vi "APPLICATION_Template.vi"(8 "error in":errorcluster) -> (0 "error out":errorcluster, 3 "Cancelled":bool)   [LabVIEW 2016]
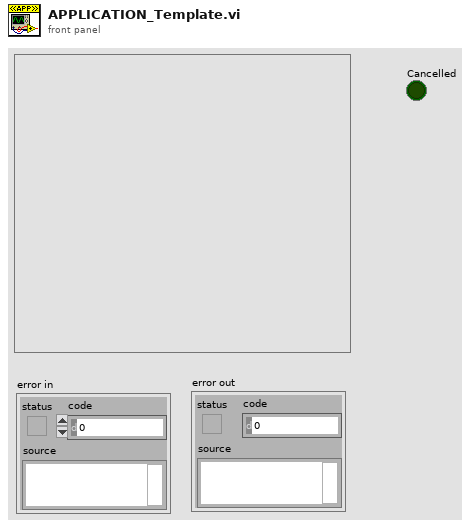
[diagram p1: front panel]
types:
  T1 = cluster{"Counter":i32, "Text":string, "Cancelled":bool}
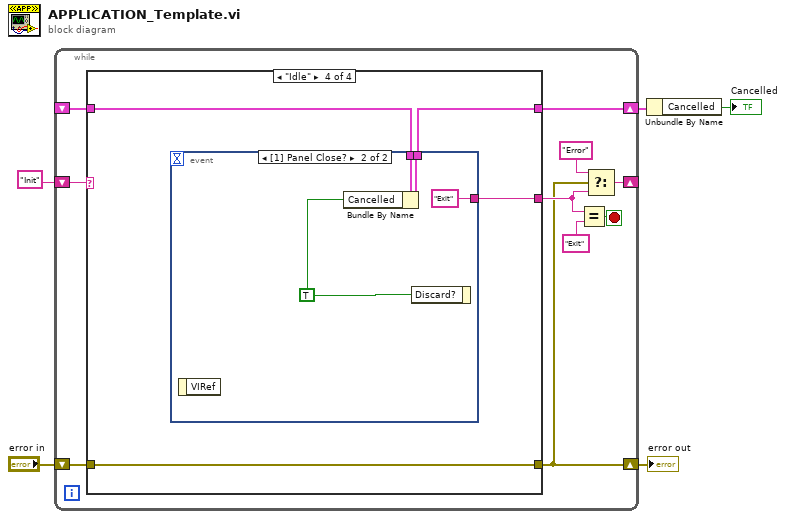
[diagram p0: block diagram]
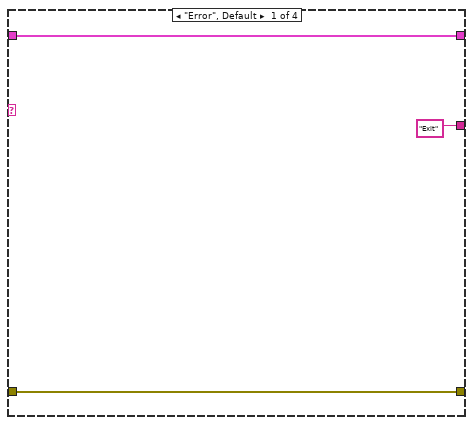
[diagram p2: hidden frame]
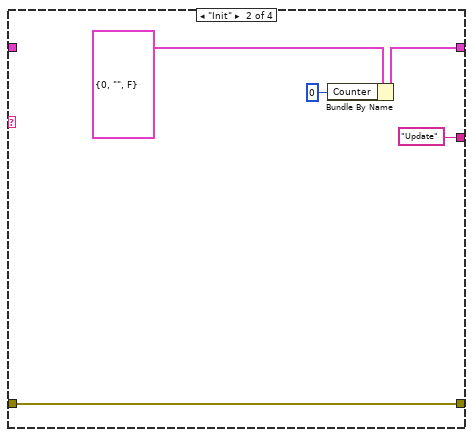
[diagram p3: hidden frame]
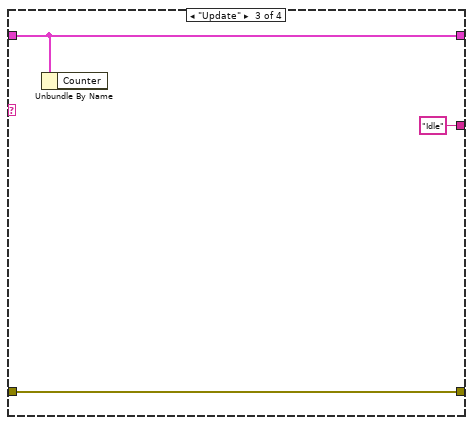
[diagram p4: hidden frame]
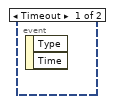
[diagram p5: hidden frame]
diagram:
  n1 = while {
    shift-right: [w8] -> w2
    shift-left: "error in" -> [w15]
    shift-right: [w13] -> _
    shift-left: "Init" -> [w14]
    shift-right: [w7] -> w3
    shift-left: _ -> [w6]
    stop <- w12 stop-if-true
    n2 = case shown="\"Idle\"" w14 {
      tunnel: w15 -> [w18 w22 w24 w27]
      tunnel: [w18 w22 w24 w27] -> w8
      tunnel: ["Exit" "Update" "Idle" w28] -> w9
      tunnel: [w16 w20 w25 w29] -> w7
      tunnel: w6 -> [w16 _ w25 w30]
      frame "Error", Default {
      }
      frame "Init" {
        n3 = Bundle By Name(cluster=T1 {"Counter"=0, "Text"="", "Cancelled"=FALSE}, "Counter"=0) -> (w20:T1)
      }
      frame "Update" {
        n4 = Unbundle By Name(w25) -> ()  [unwired: 1 out]
      }
      frame "Idle" {
        n5 = event shown="[1] Panel Close?" {
          selector: _ -> [_ _]
          dyn-events: _ -> [_ _]
          timeout: _ -> [_ _]
          tunnel: w30 -> [_ w33]
          tunnel: [_ w32] -> w29
          tunnel: [_ "Exit"] -> w28
          event Timeout {
            n6 = event-data() -> ()  [unwired: 3 out]
          }
          event Panel Close? {
            w31 = TRUE ("Discard?")
            n7 = event-data() -> ()  [unwired: 2 out]
            n8 = Bundle By Name(cluster=w33, "Cancelled"=w31) -> (w32:T1)
            n9 = event-data("Discard?"=w31) -> ()  [unwired: 1 in, 1 out]
          }
        }
      }
    }
    n10 = Equal?(x=w9, y="Exit") -> (x = y?=w12:bool)
    n11 = Select(t="Error", s=w8, f=w9) -> (s? t:f=w13:string)
  }
  "error out" <- w2
  n12 = Unbundle By Name(w3) -> ("Cancelled"=→"Cancelled":bool)
